vi "init.vi"(8 "error in":errorcluster, 10 "TBM module configuration in":refnum<class "TBM module configuration.lvclass">, 11 "FPGA Module runtime in":refnum<class "FPGA Module runtime.lvclass">) -> (0 "error out":errorcluster, 1 "data allocations":T1, 2 "execution settings":T4, 3 "FPGA Module runtime out":refnum<class "FPGA Module runtime.lvclass">)   [LabVIEW 2017, in "FPGA Module runtime.lvclass"]
doc: "Provides an interface for initializing a module at runtime. While this interface performs no operations, a child should provide an override which may open any necessary references or sessions, allocate necessary memory, and perform any final configuration validataion before providing the full configuration <b>execution data</b> to the calling process."
uses:
  FPGA Module runtime.lvclass
  <vilib>/NI/Tag Bus Module Framework/module configuration/TBM module configuration.lvclass
  <vilib>/NI/Tag Bus Module Framework/runtime/execution settings.ctl
  <vilib>/NI/Tag Bus Module Framework/channel/data tables.ctl
  <vilib>/NI/Tag Bus/dictionary/data dictionary.lvclass
  <vilib>/NI/Tag Bus/dictionary table pair.ctl
  <vilib>/NI/Tag Bus/table/data table.ctl
  configuration/FPGA Module configuration.lvclass
  <vilib>/NI/Tag Bus Module Framework/FPGA manager/methods.ctl
  configuration/FPGA Module configuration.lvclass/FPGA Module configuration.ctl
  FPGA Module runtime.lvclass/FPGA Module runtime.ctl
  configuration/Read RIO Device.vi
  <vilib>/NI/Tag Bus Module Framework/channel/TBM channel.lvclass
  <vilib>/NI/Tag Bus Module Framework/runtime/TBM module execution interface.lvclass
  <vilib>/NI/Tag Bus Module Framework/FPGA manager/FPGA manager.lvlib
  <vilib>/NI/Tag Bus/tag bus.lvlib
  <vilib>/NI/Tag Bus/table/data table.lvlib
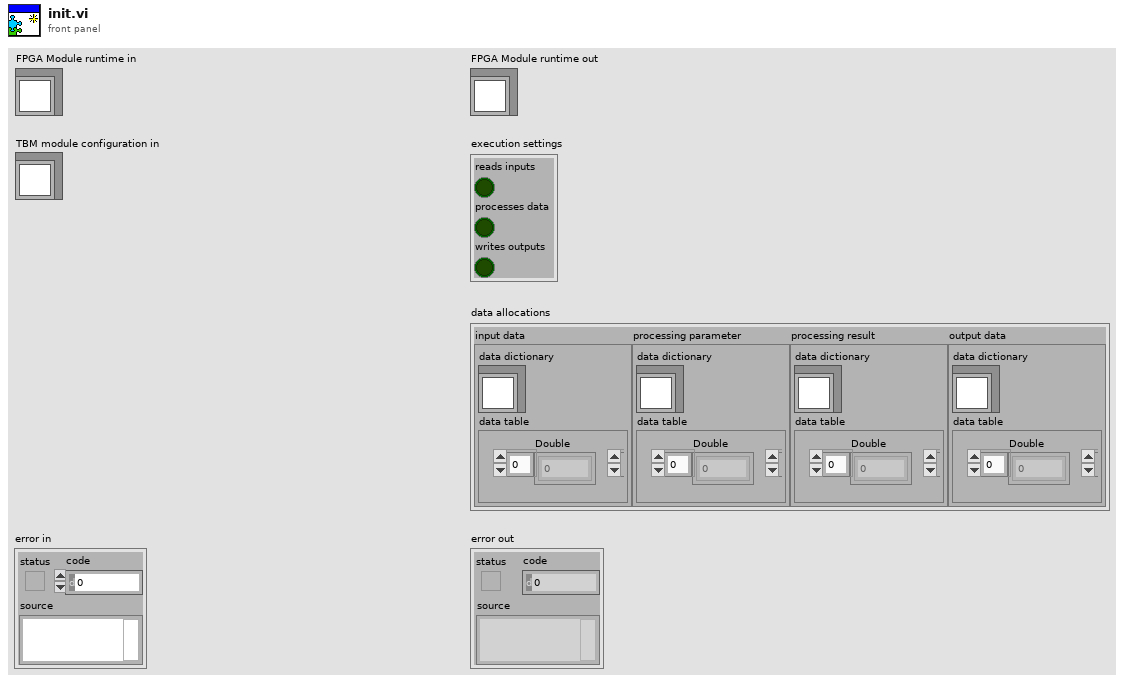
[diagram p1: front panel]
types:
  T1 = typedef "TBM channel.lvclass/data tables.ctl" = cluster{"input data":T2, "processing parameter":T2, "processing result":T2, "output data":T2}
  T2 = typedef "tag bus.lvlib/dictionary table pair.ctl" = cluster{"data dictionary":refnum<class "data dictionary.lvclass">, "data table":T3}
  T3 = typedef "tag bus.lvlib/data table.lvlib/data table.ctl" = cluster{"Double":dbl[], "Single":sgl[], "I64":i64[], "I32":i32[], "I16":i16[], "I8":i8[], "U64":u64[], "U32":u32[], "U16":u16[], "U8":u8[], "Boolean":bool[], "String":string[], "Array of Double":cluster{"DBL Array":dbl[]}[], "Array of Single":cluster{"SGL Array":sgl[]}[], "Array of I64":cluster{"I64 Array":i64[]}[], "Array of I32":cluster{"I32 Array":i32[]}[], "Array of I16":cluster{"I16 Array":i16[]}[], "Array of I8":cluster{"I8 Array":i8[]}[], "Array of U64":cluster{"U64 Array":u64[]}[], "Array of U32":cluster{"U32 Array":u32[]}[], "Array of U16":cluster{"U16 Array":u16[]}[], "Array of U8":cluster{"U8 Array":u8[]}[], "Array of Boolean":cluster{"Boolean Array":bool[]}[], "Array of String":cluster{"String Array":string[]}[]}
  T4 = typedef "TBM module execution interface.lvclass/execution settings.ctl" = cluster{"reads inputs":bool, "processes data":bool, "writes outputs":bool}
  T5 = typedef "FPGA manager.lvlib/methods.ctl" = enum16{"initialize bitfile", "cache bitfile", "locate bitfile", "close bitfile", "clear manager"}
  T6 = typedef "nirio_resource_hc.ctl" = tag
  T7 = typedef "FPGA Channel.lvclass/ControlsMappings.ctl" = cluster{"data type":T8, "fpga res type":T9[], "fpga resource":refnum<k20>[], "data indexes":i32[]}
  T8 = typedef "tag bus.lvlib/tag descriptor.lvclass/Data Type.ctl" = enum16{"Double", "Single", "I64", "I32", "I16", "I8", "U64", "U32", "U16", "U8", "Boolean", "String", "Array of Double", "Array of Single", "Array of I64", "Array of I32", "Array of I16", "Array of I8", "Array of U64", "Array of U32", "Array of U16", "Array of U8", "Array of Boolean", "Array of String"}
  T9 = typedef "FPGA Channel.lvclass/fpga resource supported data types.ctl" = enum16{"Invalid Type", "Single", "I64", "I32", "I16", "I8", "U64", "U32", "U16", "U8", "Boolean", "FXP I,20,5", "FXP I,24,5", "FXP I,24,10", "Fifo 1023,I16"}
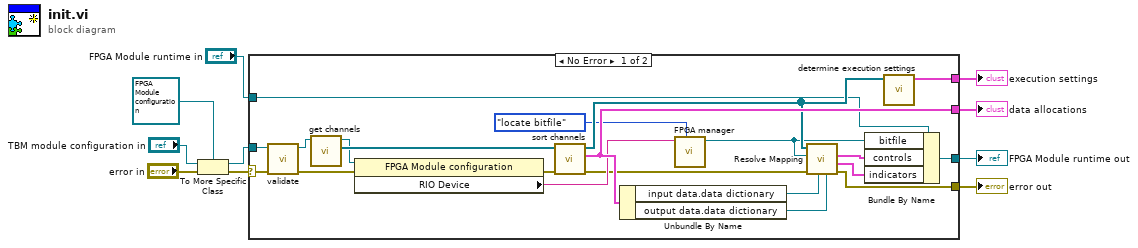
[diagram p0: block diagram]
diagram:
  n1 = To More Specific Class(target class=refnum<class "FPGA Module configuration.lvclass"> refnum ("Synchronous module configuration"), reference="TBM module configuration in", error in="error in") -> (specific class reference=w9:refnum<class "FPGA Module configuration.lvclass">, error out=w10:errorcluster)
  n2 = case shown="No Error" w10 {
    selector: w10 -> [w30 w32]
    tunnel: w9 -> [w29 _]
    tunnel: "FPGA Module runtime in" -> [w17 w33]
    tunnel: [w16 w33] -> w4
    tunnel: [w12 w32] -> w3
    tunnel: [w24 _] -> w1
    tunnel: [w31 _] -> w2
    frame No Error {
      n3 = call-dynamic "validate.vi"("error in"=w30, "FPGA Module configuration in"=w29) -> ("error out"=w19:errorcluster, "FPGA Module configuration out"=w28:refnum<class "FPGA Module configuration.lvclass">)  [unwired: 8 in]
      n4 = call-dynamic "get channels.vi"("FPGA Module configuration in"=w28) -> ("channels"=w27:refnum<class "TBM channel.lvclass">[], "FPGA Module configuration out"=w21:refnum<class "FPGA Module configuration.lvclass">)  [unwired: 9 in]
      n5 = property class="FPGA Module configuration"(reference=w21, error in=w19) -> (error out=w18:errorcluster, "RIO Device"=w20:T6)  [unwired: 1 out]
      n6 = call <vilib>:"sort channels.vi"("error in"=w18, "channels in"=w27) -> ("error out"=w13:errorcluster, "data allocations"=w24:T1, "channels out"=w23:refnum<class "TBM channel.lvclass">[])  [unwired: 7 in]
      n7 = Unbundle By Name(w24) -> ("input data.data dictionary"=w25:refnum<class "data dictionary.lvclass">, "output data.data dictionary"=w26:refnum<class "data dictionary.lvclass">)
      n8 = call <vilib>:"FPGA manager.vi"("action"=methods."locate bitfile", "RIO resource"=w20) -> ("bitfile"=w11:refnum<k20>)  [unwired: 7 in, 2 out]
      n9 = call "Resolve Mapping.vi"("output dictionary"=w26, "input dictionary"=w25, "error in"=w13, "bitfile ref"=w11, "channels in"=w23) -> ("error out"=w12:errorcluster, "indicators"=w14:T7[], "controls"=w15:T7[])  [unwired: 4 in]
      n10 = Bundle By Name(cluster=w17, "bitfile"=w11, "controls"=w15, "indicators"=w14) -> (w16:refnum<class "FPGA Module runtime.lvclass">)
      n11 = call <vilib>:"determine execution settings.vi"("channels"=w23) -> ("execution settings"=w31:T4)  [unwired: 10 in]
    }
    frame Error {
    }
  }
  "error out" <- w3
  "FPGA Module runtime out" <- w4
  "execution settings" <- w2
  "data allocations" <- w1
